vi "ColorConfig.vi"(7 "error in (no error)":errorcluster, 9 "Config":T1={"alsIntegrationTime(ms)"=10.0, "alsGain"=40, "I2C Bus"=enum."I2C On-Board", "numProximityPulses"=5, "proximityGain"=1, "proximityLEDCurrent(mA)"=50, "proximityPulseLength(ms)"=0.01, "proximitySampleTime(ms)"=10.0}, 10 "PwF_TMD37003":T3 {"Device Address" format="%.0x"}) -> (0 "error out":errorcluster, 3 "PwF_TMD37003_DevRefOut":T3 {"Device Address" format="%.0x"})   [LabVIEW 2019]
uses:
  <vilib>/Playing With Fusion Inc/Playing With Fusion Lib for FRC/PWF_TMD37003_LabVIEW/Public/TypeDefs/PwF_TMD37003_DevRef.ctl
  <vilib>/Rock Robotics/SystemInterfaces/i2clib/i2c_bus.ctl
  ArgosLib/Config/ConfigComponents/TypeDefs/Config_PwF_TMD37003.ctl
  <vilib>/Playing With Fusion Inc/Playing With Fusion Lib for FRC/PWF_TMD37003_LabVIEW/PwF_TMD37003.lvlib
  ArgosLib/ArgosLib.lvlib
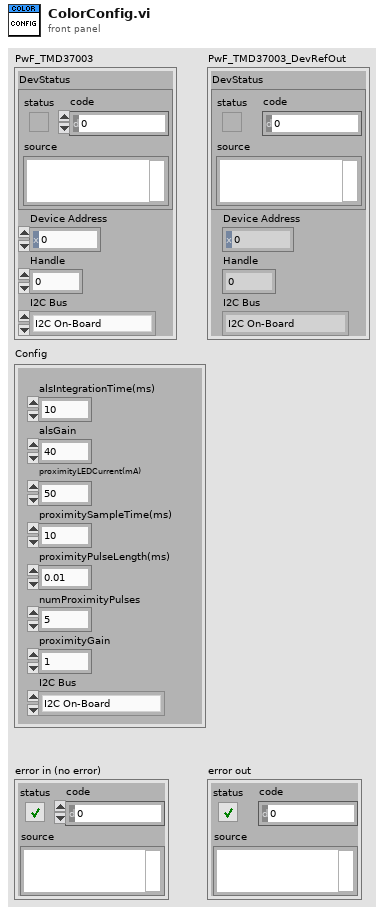
[diagram p1: front panel]
types:
  T1 = typedef "ArgosLib.lvlib/Config_PwF_TMD37003.ctl" = cluster{"alsIntegrationTime(ms)":dbl, "alsGain":u8, "I2C Bus":T2, "numProximityPulses":u8, "proximityGain":u8, "proximityLEDCurrent(mA)":u8, "proximityPulseLength(ms)":dbl, "proximitySampleTime(ms)":dbl}
  T2 = typedef "i2c_bus.ctl" = enum16{"I2C On-Board", "I2C MXP", "Invalid"}
  T3 = typedef "PlayingWithFusionLib.lvlib/PwF_TMD37003.lvlib/PwF_TMD37003_DevRef.ctl" = cluster{"DevStatus":errorcluster, "Device Address":u8, "Handle":i32, "I2C Bus":T2}
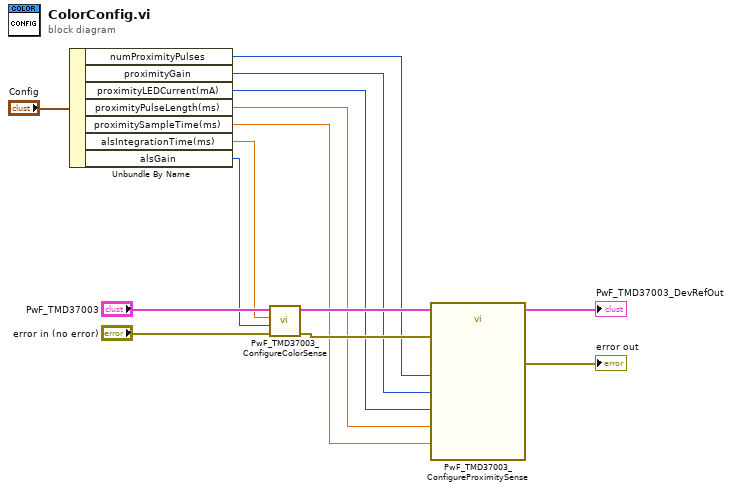
[diagram p0: block diagram]
diagram:
  n1 = Unbundle By Name("Config") -> ("numProximityPulses"=w5:u8, "proximityGain"=w4:u8, "proximityLEDCurrent(mA)"=w3:u8, "proximityPulseLength(ms)"=w2:dbl, "proximitySampleTime(ms)"=w1:dbl, "alsIntegrationTime(ms)"=w6:dbl, "alsGain"=w7:u8)
  n2 = call <vilib>:"PwF_TMD37003_ConfigureColorSense.vi"("error in (no error)"="error in (no error)", "alsGain"=w7, "alsIntegrationTime(ms)"=w6, "PwF_TMD37003_DevRefIn"="PwF_TMD37003") -> ("error out"=w13:errorcluster, "PwF_TMD37003_DevRefOut"=w10:T3)  [unwired: 6 in]
  n3 = call <vilib>:"PwF_TMD37003_ConfigureProximitySense.vi"("proximitySampleTime(ms)"=w1, "proximityLEDCurrent(mA)"=w3, "proximityPulseLength(ms)"=w2, "error in (no error)"=w13, "proximityGain"=w4, "numProximityPulses"=w5, "PwF_TMD37003_DevRefIn"=w10) -> ("error out"=→"error out":errorcluster, "PwF_TMD37003_DevRefOut"=→"PwF_TMD37003_DevRefOut":T3)  [unwired: 3 in]
